vi "DP-Online Simulplot.vi"(11 "Expt State":T1) -> ()   [LabVIEW 2020]
uses:
  <vilib>/Utility/file.llb/Write To Spreadsheet File (DBL).vi
  CFTS SubVIs/CFTS-Experiment State.ctl
panel:
  out "FileRead Errors":bool[](array[boolean])
  in  "Return":bool
  in  "Start":bool
  in  "Output Filename":string="Abel.7K"
  in  "Select F2 (0=all)":ext=16000.0
  in  "Which DP":bool=TRUE
  out "FINAL GRAPH":cluster{ext[], ext[]}[](graph)
  in  "?":ext[](array[numeric]) format="%.2f"
  out "?":string="1053-0\t15991\t-14.5\r1052-1\t15991\t-13.0\r1052-0\t15991\t-13.1\r1051-1\t15991\t-15.4\r1051-0\t15991\t-14.9\r1050-1\t15991\t-14.9\r1050-0\t15991\t-14.1\r1049-1\t15991\t-15.7\r1049-0\t15991\t-13.7\r1048-1\t15991\t-15.4\r1048-0\t15991\t-14.6\r1054-1\t15991\t-15.6\r1054-0\t15991\t-15.7\r1055-1\t15991\t-15.4\r1055-0\t15991\t-15.4\r1057-1\t15991\t-15.1\r1057-0\t15991\t-14.2\r1056-1\t15991\t-14.6\r1056-0\t15991\t-14.6\r"
  in  "LIST -  \"ID-RN;ID-RN;'":string="1058-0;1058-1;1056-0;1056-1;1057-0;1057-1;1055-0;1055-1;1054-0;1054-1;1048-0;1048-1;1049-0;1049-1;1050-0;1050-1;1051-0;1051-1;1052-0;1052-1;1053-0;"
  # "ID"
  # "f2 (Hz)"
  # "Nse Flr"
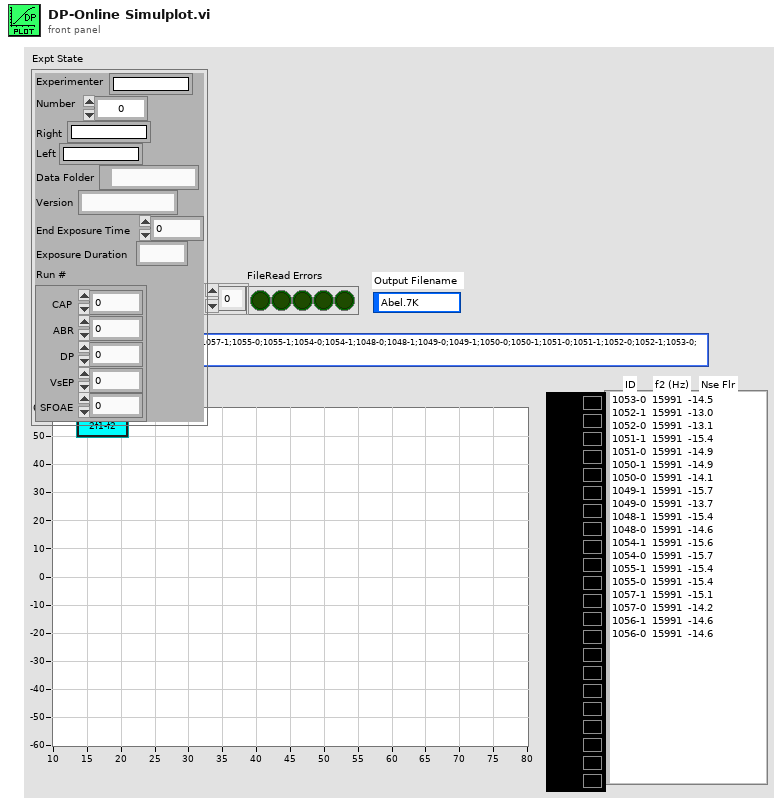
[diagram p1: front panel]
types:
  T1 = typedef "CFTS-Experiment State.ctl" = cluster{"Experimenter":string, "Number":u32, "Right":string, "Left":string, "Data Folder":path, "Version":string, "End Exposure Time":dbl, "Exposure Duration":string, "Run #":cluster{"CAP":i32, "ABR":i32, "DP":i32, "VsEP":i32, "SFOAE":i32}}
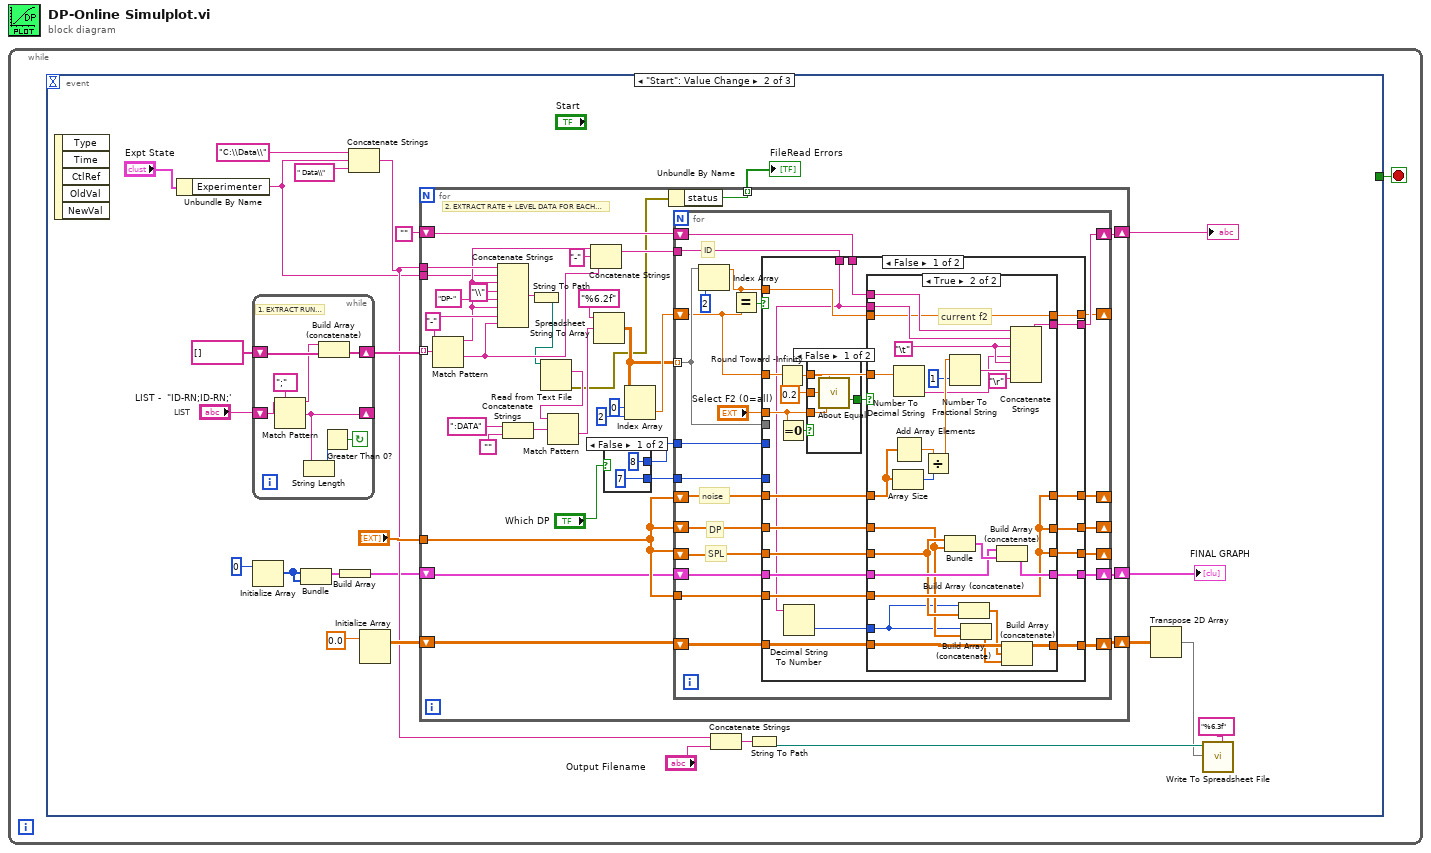
[diagram p0: block diagram]
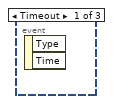
[diagram p2: hidden frame]
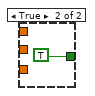
[diagram p3: hidden frame]
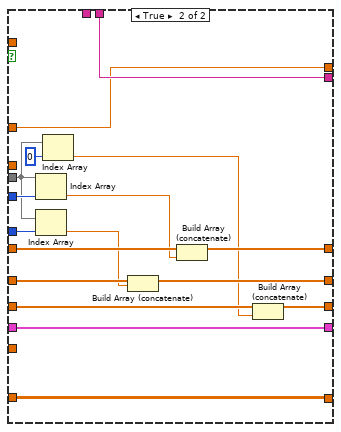
[diagram p5: hidden frame]
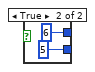
[diagram p6: hidden frame]
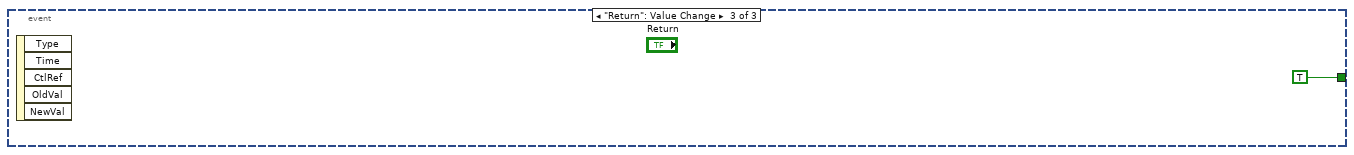
[diagram p7: hidden frame]
diagram:
  n1 = while {
    stop <- w1 stop-if-true
    n2 = event shown="[1] \"Start\": Value Change" {
      selector: _ -> [_ _ _]
      dyn-events: _ -> [_ _ _]
      timeout: _ -> [_ _ _]
      tunnel: [_ _ TRUE] -> w1
      event Timeout {
        n3 = event-data() -> ()  [unwired: 1 in, 2 out]
      }
      event "Start": Value Change {
        # "LIST"
        n4 = event-data() -> ()  [unwired: 1 in, 5 out]
        n5 = Unbundle By Name("Expt State") -> ("Experimenter"=w8:string)
        n6 = while {
          shift-left: string[] [] -> [w28]
          shift-right: [w34] -> w24
          shift-left: "LIST -  \"ID-RN;ID-RN;'" -> [w33]
          shift-right: [w29] -> _
          stop <- w31 continue-if-true
          # "1. EXTRACT RUN #S"
          n7 = Match Pattern(string=w33, regular expression=";") -> (before substring=w27:string, after substring=w29:string)  [unwired: 1 in, 2 out]
          n8 = String Length(string=w29) -> (length=w32:i32)
          n9 = Build Array (concatenate)(w27, w28) -> (w34:string[])
          n10 = Greater Than 0?(x=w32) -> (x > 0?=w31:bool)
        }
        n11 = Initialize Array(0) -> (w6:i32[])  [unwired: 1 in]
        n12 = Bundle(w6, w6) -> (w22:cluster{i32[], i32[]})  [unwired: 1 in]
        n13 = Build Array(w22) -> (w4:cluster{i32[], i32[]}[])
        n14 = Concatenate Strings("C:\\Data\\", w8, " Data\\") -> (w9:string)
        n15 = Initialize Array(0.0) -> (w20:dbl[][])  [unwired: 2 in]
        n16 = for {
          shift-right: [w60] -> w12
          shift-left: "" -> [w61]
          tunnel: "?" -> [w62]
          tunnel: w24 -> [w68] mode=indexing
          shift-right: [w57] -> w21
          shift-left: w4 -> [w58]
          tunnel: w9 -> [w56]
          shift-right: [w47] -> w14
          shift-left: w20 -> [w48]
          tunnel: w8 -> [w38]
          tunnel: [w35] -> w7 mode=indexing
          w55 = "-"
          # "2. EXTRACT RATE + LEVEL DATA FOR EACH RUN"
          n17 = Match Pattern(string=w68, regular expression=w55) -> (before substring=w50:string, after substring=w49:string)  [unwired: 1 in, 2 out]
          n18 = Concatenate Strings(w56, w38, w50, "\\", "DP-", w50, w55, w49) -> (w44:string)
          n19 = Concatenate Strings(":DATA", "") -> (w42:string)
          n20 = String To Path(string=w44) -> (path=w45:path)
          n21 = Read from Text File(file (use dialog)=w45) -> (text=w37:string, error out=w36:errorcluster)  [unwired: 3 in, 2 out]
          n22 = Match Pattern(string=w37, regular expression=w42) -> (after substring=w43:string)  [unwired: 1 in, 3 out]
          n23 = Concatenate Strings(w50, "-", w49) -> (w51:string)
          n24 = Spreadsheet String To Array(format string="%6.2f", spreadsheet string=w43) -> (array=w39:dbl[][])  [unwired: 2 in]
          n25 = case shown="False" "Which DP" {
            tunnel: [7 5] -> w66
            tunnel: [8 6] -> w67
            frame False {
            }
            frame True {
            }
          }
          n26 = Index Array(array=w39, index (row)=0, index (col)=2) -> (element=w65:dbl)
          n27 = Unbundle By Name(w36) -> ("status"=w35:bool)
          n28 = for {
            tunnel: w39 -> [w83] mode=indexing
            shift-right: [w75] -> _
            shift-left: w65 -> [w77]
            shift-right: [w89] -> _
            shift-left: w62 -> [w88]
            shift-right: [w87] -> _
            shift-left: w62 -> [w86]
            shift-right: [w85] -> _
            shift-left: w62 -> [w84]
            tunnel: w67 -> [w82]
            tunnel: w66 -> [w81]
            tunnel: w62 -> [w80]
            shift-right: [w78] -> w60
            shift-left: w61 -> [w76]
            tunnel: w51 -> [w79]
            shift-right: [w72] -> w57
            shift-left: w58 -> [w73]
            shift-right: [w69] -> w47
            shift-left: w48 -> [w70]
            # "ID"
            # "SPL"
            # "DP"
            # "noise"
            n29 = Index Array(array=w83, index=2) -> (element=w74:dbl)
            n30 = Equal?(x=w74, y=w77) -> (x = y?=w90:bool)
            n31 = case shown="False" w90 {
              tunnel: [w104 w160] -> w89
              tunnel: w88 -> [w114 w159]
              tunnel: [w105 w161] -> w87
              tunnel: w86 -> [w110 w158]
              tunnel: [w107 w162] -> w85
              tunnel: w84 -> [w111 w157]
              tunnel: w83 -> [_ w164]
              tunnel: w82 -> [_ w166]
              tunnel: w81 -> [_ w165]
              tunnel: w80 -> [w106 _]
              tunnel: [w113 w154] -> w78
              tunnel: w77 -> [w98 w153]
              tunnel: w79 -> [w94 _]
              tunnel: w76 -> [w112 w154]
              tunnel: [w103 w153] -> w75
              tunnel: w74 -> [w102 _]
              tunnel: w73 -> [w109 w152]
              tunnel: [w108 w152] -> w72
              tunnel: "Select F2 (0=all)" -> [w100 _]
              tunnel: w70 -> [w96 w151]
              tunnel: [w95 w151] -> w69
              frame False {
                n32 = Round Toward -Infinity(1:w98) -> (0:w97:dbl)
                n33 = Equal To 0?(x=w100) -> (x = 0?=w99:bool)
                n34 = Decimal String To Number(string=w94) -> (number=w93:i32)  [unwired: 2 in, 1 out]
                n35 = case shown="False" w99 {
                  tunnel: [w118 TRUE] -> w101
                  tunnel: w100 -> [w117 _]
                  tunnel: w97 -> [w116 _]
                  tunnel: 0.2 -> [w115 _]
                  frame False {
                    n36 = call "About Equal.vi"("Standard Value"=w117, "+/- Range"=w115, "Input Value"=w116) -> ("In Range?"=w118:bool)
                  }
                  frame True {
                  }
                }
                n37 = case shown="True" w101 {
                  tunnel: [w122 w140] -> w108
                  tunnel: w109 -> [w122 w139]
                  tunnel: w110 -> [_ w128]
                  tunnel: w111 -> [_ w129]
                  tunnel: w97 -> [_ w138]
                  tunnel: w112 -> [w124 w137]
                  tunnel: w94 -> [_ w136]
                  tunnel: [w124 w135] -> w113
                  tunnel: w114 -> [_ w134]
                  tunnel: [w121 w133] -> w107
                  tunnel: w106 -> [w121 w133]
                  tunnel: [w121 w133] -> w105
                  tunnel: [w121 w133] -> w104
                  tunnel: [w123 w132] -> w103
                  tunnel: w102 -> [w123 w132]
                  tunnel: w96 -> [w120 w131]
                  tunnel: [w120 w130] -> w95
                  tunnel: w93 -> [_ w127]
                  frame False {
                  }
                  frame True {
                    w145 = "\t"
                    # "current f2"
                    n38 = Array Size(array=w134) -> (size(s)=w142:i32)
                    n39 = Number To Decimal String(number=w138) -> (decimal integer string=w144:string)  [unwired: 1 in]
                    n40 = Add Array Elements(numeric array=w134) -> (sum=w141:ext)
                    n41 = Divide(x=w141, y=w142) -> (x/y=w148:ext)
                    n42 = Bundle(w129, w128) -> (w149:cluster{ext[], ext[]})  [unwired: 1 in]
                    n43 = Number To Fractional String(number=w148, precision (6)=1) -> (F-format string=w146:string)  [unwired: 2 in]
                    n44 = Build Array (concatenate)(w127, w129) -> (w126:ext[])
                    n45 = Build Array (concatenate)(w127, w128) -> (w125:ext[])
                    n46 = Build Array (concatenate)(w139, w149) -> (w140:cluster{ext[], ext[]}[])
                    n47 = Build Array (concatenate)(w131, w126, w125) -> (w130:ext[][])
                    n48 = Concatenate Strings(w137, w136, w145, w144, w145, w146, "\r") -> (w135:string)
                  }
                }
              }
              frame True {
                n49 = Index Array(array=w164, index=w166) -> (element=w155:dbl)
                n50 = Index Array(array=w164, index=w165) -> (element=w150:dbl)
                n51 = Index Array(array=w164, index=0) -> (element=w156:dbl)
                n52 = Build Array (concatenate)(w158, w150) -> (w161:ext[])
                n53 = Build Array (concatenate)(w159, w155) -> (w160:ext[])
                n54 = Build Array (concatenate)(w157, w156) -> (w162:ext[])
              }
            }
          }
        }
        "FINAL GRAPH" <- w21
        "?" <- w12
        "FileRead Errors" <- w7
        n55 = Concatenate Strings(w9, "Output Filename") -> (w17:string)
        n56 = String To Path(string=w17) -> (path=w16:path)
        n57 = Transpose 2D Array(2D array=w14) -> (transposed array=w13:ext[][])
        n58 = call-poly <vilib>:"Write To Spreadsheet File.vi"("format (%.3f)"="%6.3f", "2D data"=w13, "file path (dialog if empty)"=w16) -> ()  [unwired: 5 in, 1 out]
      }
      event "Return": Value Change {
        n59 = event-data() -> ()  [unwired: 1 in, 5 out]
      }
    }
  }
